vi "Update Main FP Controls.vi"(8 "error in (no error)":errorcluster, 11 "dialog info in":T1={"steering frame ref"=refnum, "active wheel indexes"=[], "FP Refs"={"VI Refnum"=refnum, "Menu Ref"=refnum, "Sub Panel"=refnum, "picture"=refnum, "Steering Type"=refnum, "zoom in"=refnum, "zoom out"=refnum, "zoom extents"=refnum, "Wheels"=refnum, "Add Wheel"=refnum, "Remove Wheel"=refnum, "Copy Wheel"=refnum, "Angle Units"=refnum}, "subpanel info"={"subpanel VI refs"=[], "subpanel types"=[], "main to subpanel command events"=[]}, "picture dragging state"={"dragging"=FALSE, "wheel index"=-1, "dragging mode"=enum."translate", "wheel start position"={"x"=0.0, "y"=0.0, "theta"=0.0}, "relative mouse position"={"x"=0.0, "y"=0.0}, "relative mouse init angle (rad)"=0.0}, "picture size (pixels)"={"Width"=500, "Height"=500}, "picture grid"=bytes[0], "click zones group"={"click zones array"=[], "num click zones"=0}, "draw options"={"draw wheel states?"=FALSE, "highlight wheel index"=-1, "pixels per unit"=10.0, "draw forward velocity?"=FALSE, "velocity scale"=1.0}}) -> (0 "error out":errorcluster, 3 "dialog info out":T1={"steering frame ref"=refnum, "active wheel indexes"=[], "FP Refs"={"VI Refnum"=refnum, "Menu Ref"=refnum, "Sub Panel"=refnum, "picture"=refnum, "Steering Type"=refnum, "zoom in"=refnum, "zoom out"=refnum, "zoom extents"=refnum, "Wheels"=refnum, "Add Wheel"=refnum, "Remove Wheel"=refnum, "Copy Wheel"=refnum, "Angle Units"=refnum}, "subpanel info"={"subpanel VI refs"=[], "subpanel types"=[], "main to subpanel command events"=[]}, "picture dragging state"={"dragging"=FALSE, "wheel index"=-1, "dragging mode"=enum."translate", "wheel start position"={"x"=0.0, "y"=0.0, "theta"=0.0}, "relative mouse position"={"x"=0.0, "y"=0.0}, "relative mouse init angle (rad)"=0.0}, "picture size (pixels)"={"Width"=500, "Height"=500}, "picture grid"=bytes[0], "click zones group"={"click zones array"=[], "num click zones"=0}, "draw options"={"draw wheel states?"=FALSE, "highlight wheel index"=-1, "pixels per unit"=10.0, "draw forward velocity?"=FALSE, "velocity scale"=1.0}})   [LabVIEW 2017, in "NI_Robotics_Configure Steering Frame.lvlib"]
uses:
  <vilib>/robotics/Dialog/Configure Steering Frame/NI_Robotics_Configure Steering Frame.lvlib
  <vilib>/robotics/Dialog/Configure Steering Frame/Dialog Info.ctl
  <vilib>/robotics/Steering/Steering Frame/NI_Robotics_Steering Frame.lvclass
  <vilib>/robotics/Dialog/Configure Steering Frame/FP Refs.ctl
  <vilib>/robotics/Dialog/Configure Steering Frame/Subpanel Info.ctl
  <vilib>/robotics/Dialog/Configure Steering Frame/Main to Subpanel Command Event.ctl
  <vilib>/robotics/Dialog/Configure Steering Frame/Main to Subpanel Command.ctl
  <vilib>/robotics/Dialog/Configure Steering Frame/Dragging State.ctl
  <vilib>/robotics/Dialog/Configure Steering Frame/Dragging Mode.ctl
  <vilib>/Utility/miscctls.llb/LVBoundsTypeDef.ctl
  <vilib>/robotics/Dialog/Configure Steering Frame/Click Zone.ctl
  <vilib>/robotics/Utilities/Visualization/Steering Visualization/Steering Picture/Draw Steering Frame Options.ctl
  <vilib>/robotics/Dialog/Configure Steering Frame/Steering Type.ctl
  <vilib>/robotics/Steering/Steering Frame/NI_Robotics_Steering Frame.lvclass/NI_Robotics_Steering Frame.ctl
  <vilib>/robotics/Steering/Wheel/NI_Robotics_Wheel.lvclass/NI_Robotics_Wheel.ctl
  <vilib>/robotics/Steering/Steering Frame/Get Multiple Wheels in Steering Frame.vi
  <vilib>/robotics/Steering/Wheel/NI_Robotics_Wheel.lvclass
  <vilib>/robotics/Utilities/Visualization/Steering Visualization/Steering Picture/NI_Robotics_Steering Picture.lvlib
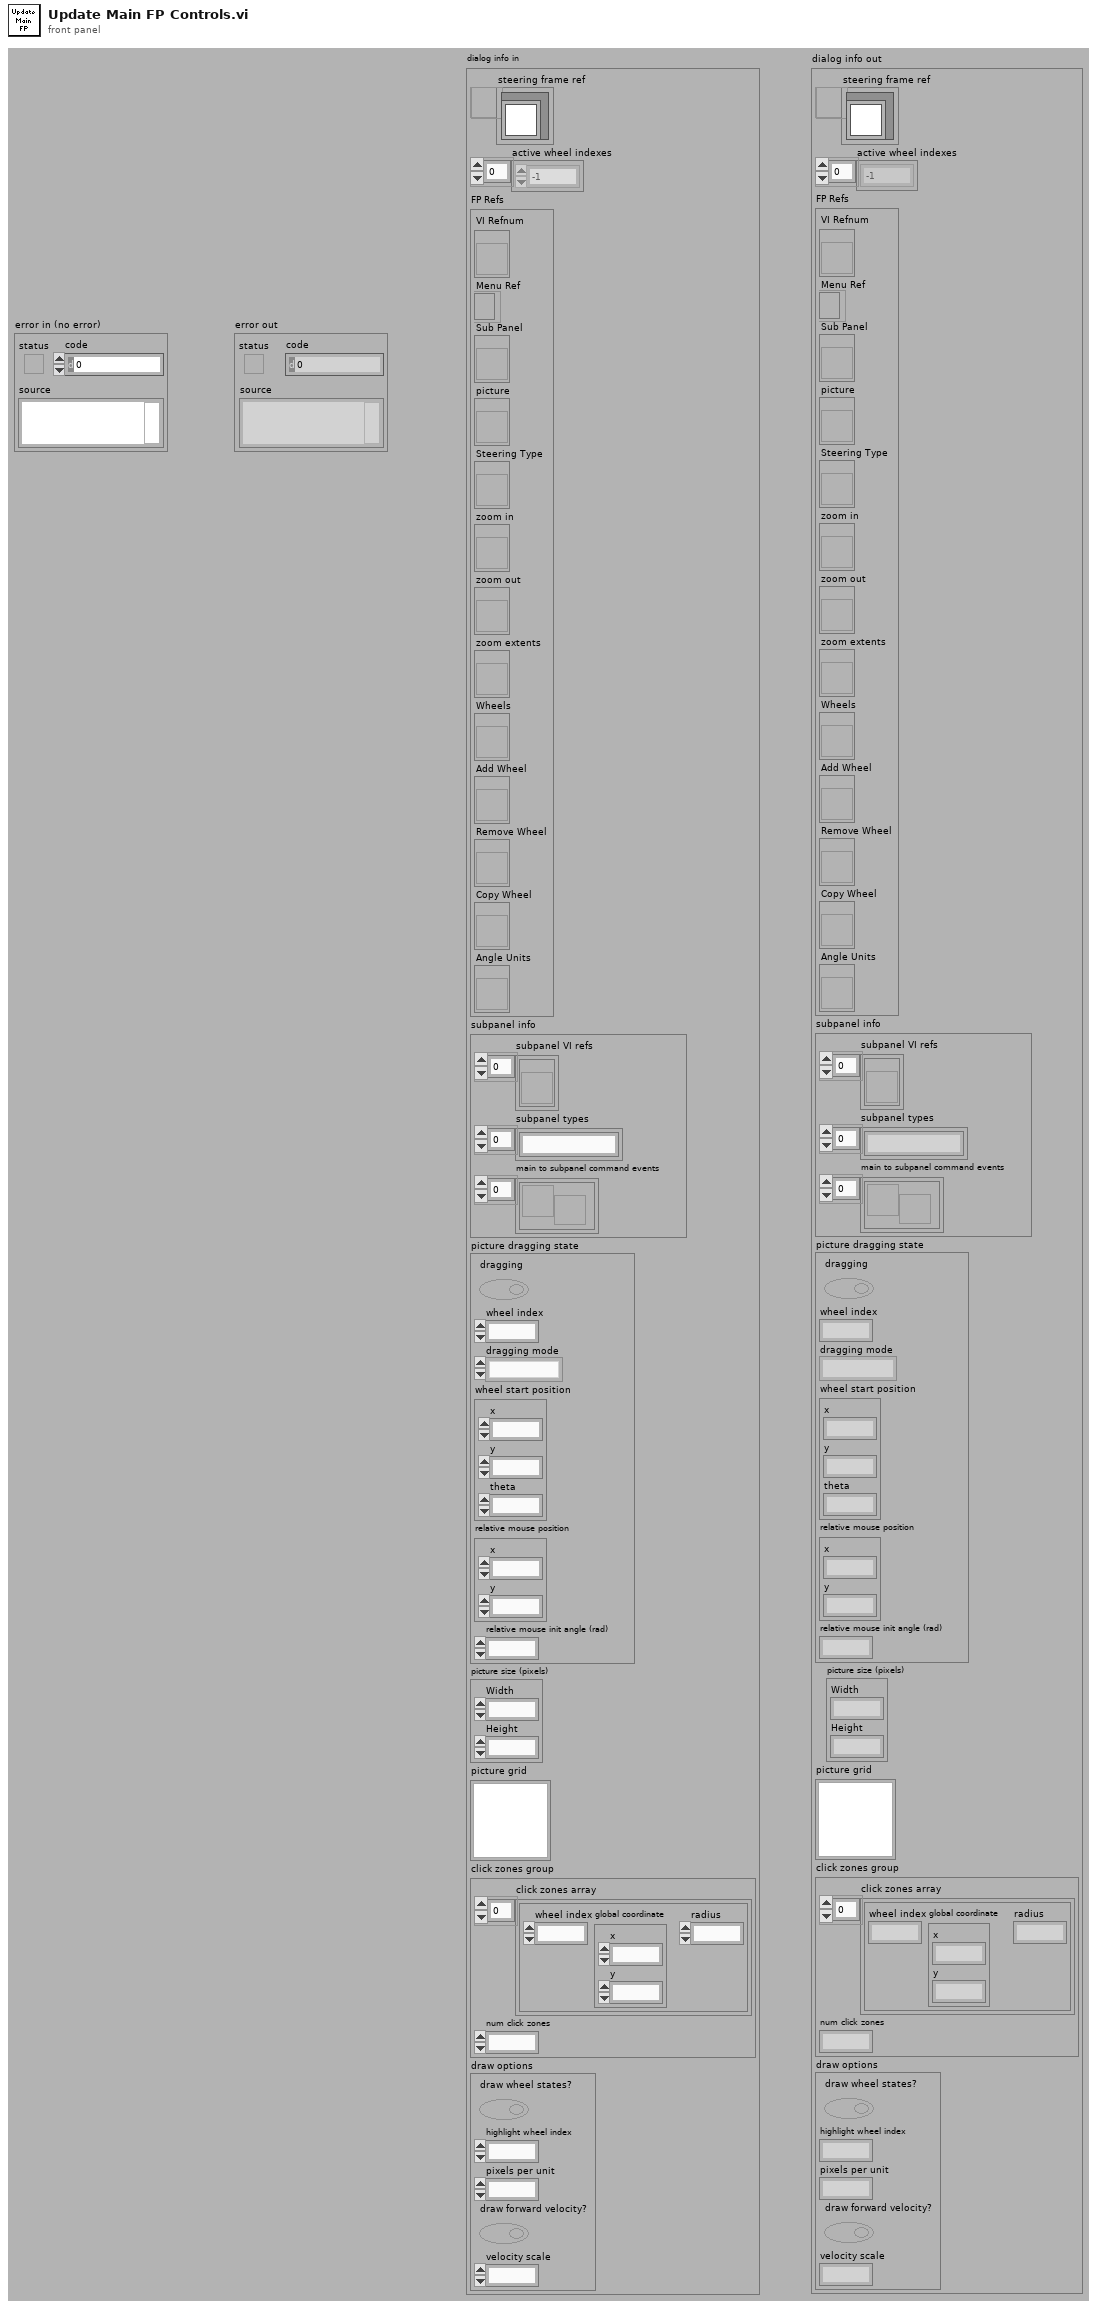
[diagram p1: front panel]
types:
  T1 = typedef "NI_Robotics_Configure Steering Frame.lvlib/Dialog Info.ctl" = cluster{"steering frame ref":refnum<data-value>, "active wheel indexes":i32[], "FP Refs":T2, "subpanel info":T3, "picture dragging state":T5, "picture size (pixels)":T7, "picture grid":picture, "click zones group":cluster{"click zones array":T8[], "num click zones":i32}, "draw options":T9}
  T2 = typedef "NI_Robotics_Configure Steering Frame.lvlib/FP Refs.ctl" = cluster{"VI Refnum":refnum<vi>, "Menu Ref":refnum<k9>, "Sub Panel":refnum<vi>, "picture":refnum<vi>, "Steering Type":refnum<vi>, "zoom in":refnum<vi>, "zoom out":refnum<vi>, "zoom extents":refnum<vi>, "Wheels":refnum<vi>, "Add Wheel":refnum<vi>, "Remove Wheel":refnum<vi>, "Copy Wheel":refnum<vi>, "Angle Units":refnum<vi>}
  T3 = typedef "NI_Robotics_Configure Steering Frame.lvlib/Subpanel Info.ctl" = cluster{"subpanel VI refs":refnum<vi>[], "subpanel types":string[], "main to subpanel command events":T4[]}
  T4 = typedef "NI_Robotics_Configure Steering Frame.lvlib/Main to Subpanel Command Event.ctl" = refnum<user-event>
  T5 = typedef "NI_Robotics_Configure Steering Frame.lvlib/Dragging State.ctl" = cluster{"dragging":bool, "wheel index":i32, "dragging mode":T6, "wheel start position":cluster{"x":dbl, "y":dbl, "theta":dbl}, "relative mouse position":cluster{"x":dbl, "y":dbl}, "relative mouse init angle (rad)":dbl}
  T6 = typedef "NI_Robotics_Configure Steering Frame.lvlib/Dragging Mode.ctl" = enum16{"translate", "rotate"}
  T7 = typedef "LVBoundsTypeDef.ctl" = cluster{"Width":u32, "Height":u32}
  T8 = typedef "NI_Robotics_Configure Steering Frame.lvlib/Click Zone.ctl" = cluster{"wheel index":i32, "global coordinate":cluster{"x":dbl, "y":dbl}, "radius":dbl}
  T9 = typedef "NI_Robotics_Steering Picture.lvlib/Draw Steering Frame Options.ctl" = cluster{"draw wheel states?":bool, "highlight wheel index":i32, "pixels per unit":dbl, "draw forward velocity?":bool, "velocity scale":dbl}
  T10 = enum8{"Enabled", "Disabled", "Disabled and Grayed Out"}
  T11 = typedef "NI_Robotics_Configure Steering Frame.lvlib/Steering Type.ctl" = u16
  T12 = typedef "NI_Robotics_Configure Steering Frame.lvlib/Angle Mode.ctl" = u16
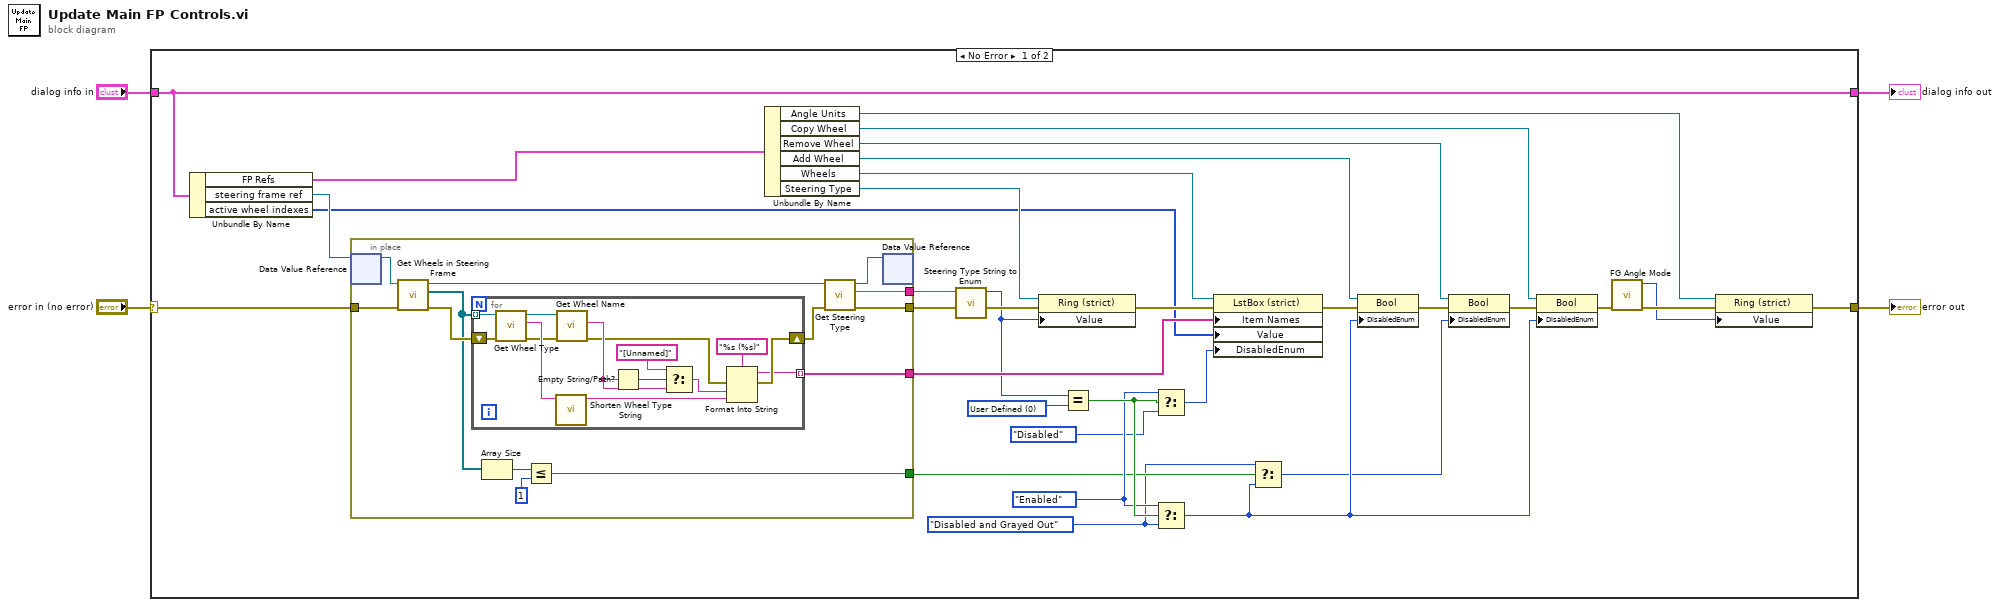
[diagram p0: block diagram]
diagram:
  n1 = case shown="No Error" "error in (no error)" {
    selector: "error in (no error)" -> [w33 w65]
    tunnel: [w15 w65] -> w3
    tunnel: "dialog info in" -> [w35 w64]
    tunnel: [w35 w64] -> w1
    frame No Error {
      w7 = T10."Disabled and Grayed Out" ("Disabled")
      w11 = T10."Enabled" ("Disabled")
      w24 = T11 0 items=["User Defined", "Differential", "Ackermann", "Mecanum"] ("y")
      n2 = Unbundle By Name(w35) -> ("FP Refs"=w36:T2, "steering frame ref"=w34:refnum<data-value>, "active wheel indexes"=w26:i32[])
      n3 = in-place {
        in-place-border: [w48] -> w31
        in-place-border: w33 -> [w44]
        in-place-border: [w47] -> w32
        in-place-border: [w41] -> w27
        in-place-border: [w37] -> w8
        n4 = in-place-dvr #1(w34) -> (w46:refnum<class "NI_Robotics_Steering Frame.lvclass">)  [unwired: 1 out]
        n5 = call-poly <vilib>:"Get Wheels in Steering Frame.vi"("error in (no error)"=w44, "steering frame in"=w46) -> ("error out"=w43:errorcluster, "wheels"=w40:refnum<class "NI_Robotics_Wheel.lvclass">[], "steering frame out"=w45:refnum<class "NI_Robotics_Steering Frame.lvclass">)  [unwired: 3 in, 4 out]
        n6 = for {
          tunnel: w40 -> [w53] mode=indexing
          shift-right: [w51] -> w42
          shift-left: w43 -> [w52]
          tunnel: [w50] -> w41 mode=indexing
          n7 = call-dynamic "Get Wheel Type.vi"("error in (no error)"=w52, "wheel in"=w53) -> ("error out"=w56:errorcluster, "wheel type"=w62:string, "wheel out"=w55:refnum<class "NI_Robotics_Wheel.lvclass">)  [unwired: 7 in]
          n8 = call <vilib>:"Shorten Wheel Type String.vi"("wheel type"=w62) -> ("short wheel type"=w63:string)  [unwired: 10 in]
          n9 = call <vilib>:"Get Wheel Name.vi"("error in (no error)"=w56, "wheel in"=w55) -> ("error out"=w57:errorcluster, "wheel name"=w59:string)  [unwired: 7 in, 1 out]
          n10 = Empty String/Path?(string/path=w59) -> (empty?=w58:bool)
          n11 = Select(t="[Unnamed]" ("format string"), s=w58, f=w59) -> (s? t:f=w60:string)
          n12 = Format Into String(format string="%s (%s)", error in=w57, w60, w63) -> (resulting string=w50:string, error out=w51:errorcluster)  [unwired: 1 in]
        }
        n13 = Array Size(array=w40) -> (size(s)=w39:i32)
        n14 = Less Or Equal?(x=w39, y=1) -> (x <= y?=w37:bool)
        n15 = call-dynamic "Get Steering Type.vi"("error in (no error)"=w42, "steering frame in"=w45) -> ("error out"=w48:errorcluster, "steering type"=w47:string, "steering frame out"=w49:refnum<class "NI_Robotics_Steering Frame.lvclass">)  [unwired: 7 in]
        n16 = in-place-dvr #1(w49) -> ()  [unwired: 2 out]
      }
      n17 = Unbundle By Name(w36) -> ("Angle Units"=w13:refnum<vi>, "Copy Wheel"=w18:refnum<vi>, "Remove Wheel"=w19:refnum<vi>, "Add Wheel"=w22:refnum<vi>, "Wheels"=w29:refnum<vi>, "Steering Type"=w30:refnum<vi>)
      n18 = call <vilib>:"Steering Type String to Enum.vi"("steering type_string"=w32) -> ("steering type_enum"=w25:T11)  [unwired: 9 in, 1 out]
      n19 = property class="Ring (strict)"(reference=w30, error in=w31, "Value"=w25) -> (error out=w28:errorcluster)  [unwired: 1 out]
      n20 = Equal?(x=w25, y=w24) -> (x = y?=w12:bool)
      n21 = Select(t=w11, s=w12, f=T10."Disabled" ("Disabled")) -> (s? t:f=w9:T10)
      n22 = Select(t=w11, s=w12, f=w7) -> (s? t:f=w6:T10)
      n23 = property class="LstBox (strict)"(reference=w29, error in=w28, "Item Names"=w27, "Value"=w26, "DisabledEnum"=w9) -> (error out=w23:errorcluster)  [unwired: 1 out]
      n24 = Select(t=w7, s=w8, f=w6) -> (s? t:f=w5:T10)
      n25 = property class="Bool"(reference=w22, error in=w23, "DisabledEnum"=w6) -> (error out=w21:errorcluster)  [unwired: 1 out]
      n26 = property class="Bool"(reference=w19, error in=w21, "DisabledEnum"=w5) -> (error out=w20:errorcluster)  [unwired: 1 out]
      n27 = property class="Bool"(reference=w18, error in=w20, "DisabledEnum"=w6) -> (error out=w17:errorcluster)  [unwired: 1 out]
      n28 = call <vilib>:"FG Angle Mode.vi"("error in (no error)"=w17) -> ("error out"=w16:errorcluster, "angle mode out"=w14:T12)  [unwired: 9 in]
      n29 = property class="Ring (strict)"(reference=w13, error in=w16, "Value"=w14) -> (error out=w15:errorcluster)  [unwired: 1 out]
    }
    frame Error {
    }
  }
  "error out" <- w3
  "dialog info out" <- w1
